vi "Permissions to Bit Mask.vi"(1 "Permissions":T1) -> (0 "Bit Mask":u32 format="%.0o")   [LabVIEW 2021, in "Field_RnD_Services_LIBSSH2_Toolkit.lvlib"]
doc: "Converts the POSIX-style permissions to a bit mask-based mode."
uses:
  Field_RnD_Services_LIBSSH2_Toolkit.lvlib
  Type Definitions/Permissions.ctl
  Type Definitions/Modes.ctl
  Type Definitions/Bit Mask Modes.ctl
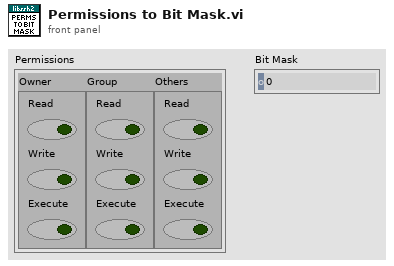
[diagram p1: front panel]
types:
  T1 = typedef "Field_RnD_Services_LIBSSH2_Toolkit.lvlib/Permissions.ctl" = cluster{"Owner":T2, "Group":T2, "Others":T2}
  T2 = typedef "Field_RnD_Services_LIBSSH2_Toolkit.lvlib/Modes.ctl" = cluster{"Read":bool, "Write":bool, "Execute":bool}
  T3 = typedef "Field_RnD_Services_LIBSSH2_Toolkit.lvlib/Bit Mask Modes.ctl" = u32
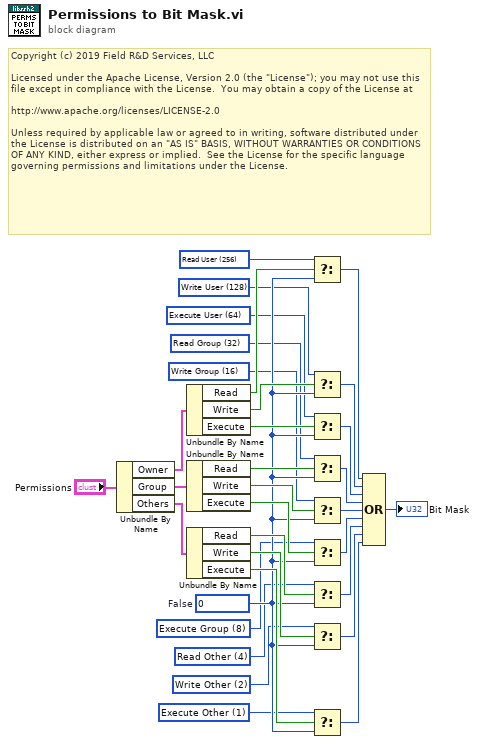
[diagram p0: block diagram]
diagram:
  w1 = T3 1 items=["Read User"=256, "Write User"=128, "Execute User"=64, "Read Group"=32, "Write Group"=16, "Execute Group"=8, "Read Other"=4, "Write Other"=2, "Execute Other"=1] ("Bit Mask Mode")
  w2 = T3 2 items=["Read User"=256, "Write User"=128, "Execute User"=64, "Read Group"=32, "Write Group"=16, "Execute Group"=8, "Read Other"=4, "Write Other"=2, "Execute Other"=1] ("Bit Mask Mode")
  w3 = T3 4 items=["Read User"=256, "Write User"=128, "Execute User"=64, "Read Group"=32, "Write Group"=16, "Execute Group"=8, "Read Other"=4, "Write Other"=2, "Execute Other"=1] ("Bit Mask Mode")
  w4 = T3 8 items=["Read User"=256, "Write User"=128, "Execute User"=64, "Read Group"=32, "Write Group"=16, "Execute Group"=8, "Read Other"=4, "Write Other"=2, "Execute Other"=1] ("Bit Mask Mode")
  w5 = T3 16 items=["Read User"=256, "Write User"=128, "Execute User"=64, "Read Group"=32, "Write Group"=16, "Execute Group"=8, "Read Other"=4, "Write Other"=2, "Execute Other"=1] ("Bit Mask Mode")
  w6 = T3 32 items=["Read User"=256, "Write User"=128, "Execute User"=64, "Read Group"=32, "Write Group"=16, "Execute Group"=8, "Read Other"=4, "Write Other"=2, "Execute Other"=1] ("Bit Mask Mode")
  w7 = T3 64 items=["Read User"=256, "Write User"=128, "Execute User"=64, "Read Group"=32, "Write Group"=16, "Execute Group"=8, "Read Other"=4, "Write Other"=2, "Execute Other"=1] ("Bit Mask Mode")
  w8 = T3 128 items=["Read User"=256, "Write User"=128, "Execute User"=64, "Read Group"=32, "Write Group"=16, "Execute Group"=8, "Read Other"=4, "Write Other"=2, "Execute Other"=1] ("Bit Mask Mode")
  w9 = T3 256 items=["Read User"=256, "Write User"=128, "Execute User"=64, "Read Group"=32, "Write Group"=16, "Execute Group"=8, "Read Other"=4, "Write Other"=2, "Execute Other"=1] ("Bit Mask Mode")
  w20 = u32 0  # False
  # "Copyright (c) 2019 Field R&D Services, LLC\n\nLicensed under the Apache License, Version 2.0 (the \"License\"); you may not use this file except in compliance with the License.  You may obtain a copy of the License at\n\nhttp://www.apache.org/licenses/LICENSE-2.0\n\nUnless required by applicable law or agreed to in writing, software distributed under the License is distributed on an \"AS IS\" BASIS, WITHOUT WARRANTIES OR CONDITIONS OF ANY KIND, either express or implied.  See the License for the specific language governing permissions and limitations under the License."
  n1 = Unbundle By Name("Permissions") -> ("Owner"=w32:T2, "Group"=w31:T2, "Others"=w30:T2)
  n2 = Unbundle By Name(w32) -> ("Read"=w29:bool, "Write"=w28:bool, "Execute"=w27:bool)
  n3 = Unbundle By Name(w31) -> ("Read"=w26:bool, "Write"=w25:bool, "Execute"=w24:bool)
  n4 = Unbundle By Name(w30) -> ("Read"=w23:bool, "Write"=w22:bool, "Execute"=w21:bool)
  n5 = Select(t=w9, s=w29, f=w20) -> (s? t:f=w19:T3)
  n6 = Select(t=w8, s=w28, f=w20) -> (s? t:f=w18:T3)
  n7 = Select(t=w7, s=w27, f=w20) -> (s? t:f=w17:T3)
  n8 = Select(t=w6, s=w26, f=w20) -> (s? t:f=w16:T3)
  n9 = Select(t=w5, s=w25, f=w20) -> (s? t:f=w15:T3)
  n10 = Select(t=w4, s=w24, f=w20) -> (s? t:f=w14:T3)
  n11 = Select(t=w3, s=w23, f=w20) -> (s? t:f=w13:T3)
  n12 = Select(t=w2, s=w22, f=w20) -> (s? t:f=w12:T3)
  n13 = Select(t=w1, s=w21, f=w20) -> (s? t:f=w11:T3)
  n14 = Compound Arithmetic op=OR(w19, w18, w17, w16, w15, w14, w13, w12, w11) -> (→"Bit Mask":T3)
